vi "CalculateFrames.vi"(8 "Program Spin Coater\nSpeed (rpm)          Time (s)":dbl[][](array[numeric]), 9 "Seconds End":dbl[unit], 10 "Seconds Start":dbl[unit], 11 "Frame Rate":dbl[unit]) -> (1 "Time":dbl, 2 "Frames":i32)   [LabVIEW 2020]
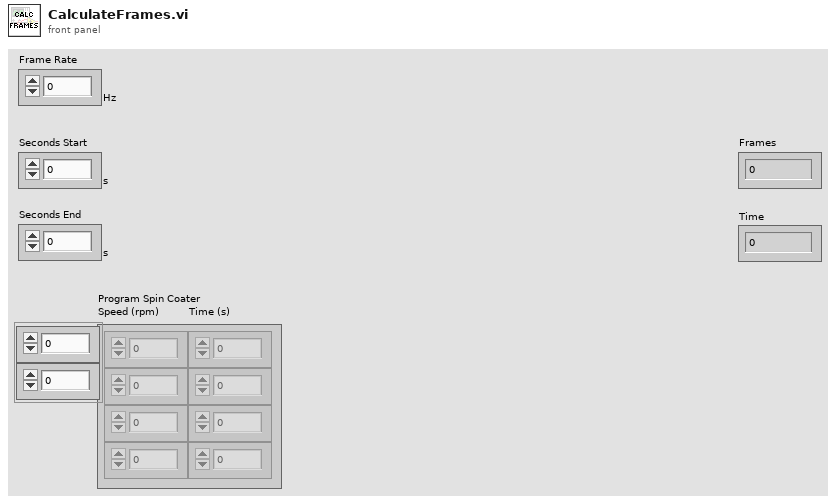
[diagram p1: front panel]
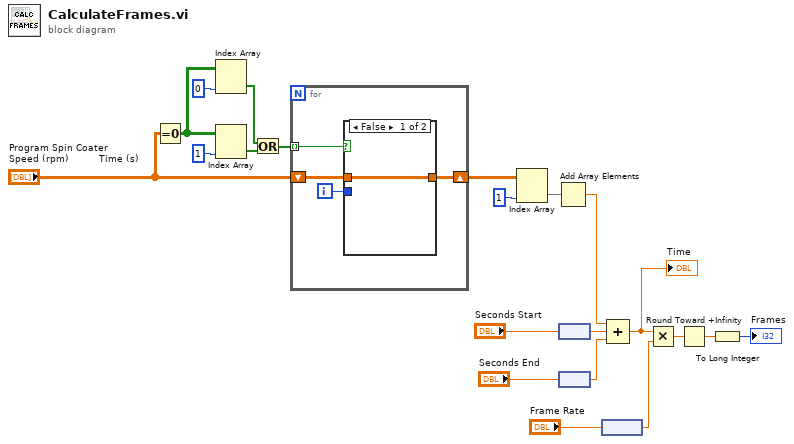
[diagram p0: block diagram]
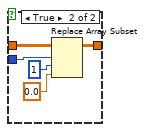
[diagram p2: hidden frame]
diagram:
  n1 = Equal To 0?(x="Program Spin Coater\nSpeed (rpm)          Time (s)") -> (x = 0?=w20:bool[][])
  n2 = Index Array(array=w20, index (col)=0 ("disabled index (col)")) -> (element=w18:bool[])  [unwired: 1 in]
  n3 = Index Array(array=w20, index (col)=1 ("disabled index (col)")) -> (element=w17:bool[])  [unwired: 1 in]
  n4 = Or(x=w18, y=w17) -> (x .or. y?=w16:bool[])
  n5 = for {
    tunnel: w16 -> [w24] mode=indexing
    shift-right: [w22] -> w14
    shift-left: "Program Spin Coater\nSpeed (rpm)          Time (s)" -> [w25]
    i -> [w23]
    n6 = case shown="False" w24 {
      tunnel: w25 -> [w26 w31]
      tunnel: w23 -> [_ w30]
      tunnel: [w26 w27] -> w22
      frame False {
      }
      frame True {
        n7 = Replace Array Subset(array=w31, new element=0.0 ("new element/subarray"), index (row)=w30, index (col)=1 ("disabled index (col)")) -> (w27:dbl[][])
      }
    }
  }
  n8 = Index Array(array=w14, index (col)=1 ("disabled index (col)")) -> (element=w12:dbl[])  [unwired: 1 in]
  n9 = Add Array Elements(numeric array=w12) -> (sum=w11:dbl)
  n10 = node("Seconds Start") -> (w9:dbl)
  n11 = node("Seconds End") -> (w7:dbl)
  n12 = node("Frame Rate") -> (w4:dbl)
  n13 = Compound Arithmetic op=ADD(w11, w9, w7) -> (w6:dbl)
  "Time" <- w6
  n14 = Multiply(x=w6, y=w4) -> (x*y=w3:dbl)
  n15 = Round Toward +Infinity(x=w3) -> (ceil(x): smallest int >= x=w2:dbl)
  n16 = To Long Integer(number=w2) -> (32bit integer=→"Frames":i32)
